vi "Koloruj wskazniki.vi"(4 "Kolor High":u32(colorbox)=16711680, 5 "High":bool, 6 "Kolor Low":u32(colorbox)=16860, 7 "Low":bool, 8 "error in (no error)":errorcluster, 11 "AI Refnum":refnum<vi>) -> (0 "error out":errorcluster)   [LabVIEW 2014]
doc: "Koloruje wskaźnik kanału analogowego nad panelem\nw zależności od zakresu ADC w zakresie/za wysoko/za nisko"
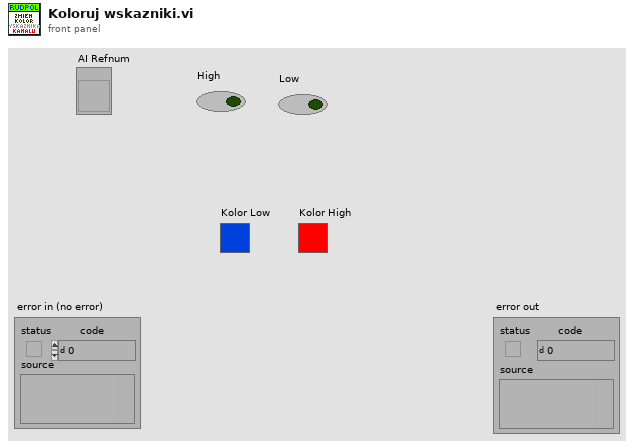
[diagram p1: front panel]
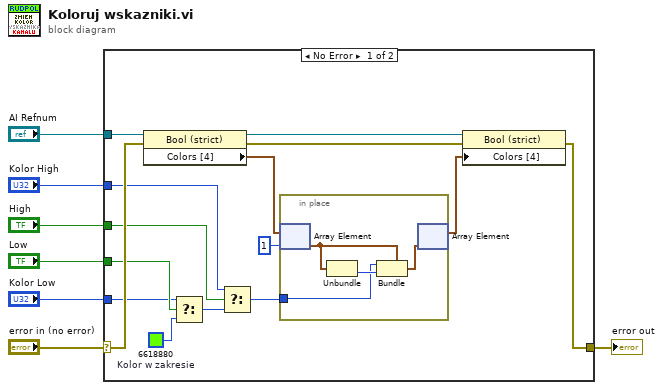
[diagram p0: block diagram]
diagram:
  n1 = case shown="No Error" "error in (no error)" {
    selector: "error in (no error)" -> [w20 w27]
    tunnel: [w19 w27] -> w6
    tunnel: "AI Refnum" -> [w22 _]
    tunnel: "Kolor Low" -> [w13 _]
    tunnel: "Kolor High" -> [w8 _]
    tunnel: "Low" -> [w14 _]
    tunnel: "High" -> [w11 _]
    frame No Error {
      w12 = u32 6618880  # Kolor w zakresie
      n2 = property class="Bool (strict)"(reference=w22, error in=w20) -> (reference out=w21:refnum<vi>, error out=w18:errorcluster, "Colors [4]"=w17:cluster{u32, u32}[])
      n3 = Select(t=w13, s=w14, f=w12) -> (s? t:f=w10:u32)
      n4 = Select(t=w8, s=w11, f=w10) -> (s? t:f=w9:u32)
      n5 = in-place {
        in-place-border: w9 -> [w23]
        n6 = in-place-array #1(w17, 1) -> (w25:cluster{u32, u32})
        n7 = Unbundle(w25) -> (w24:u32)  [unwired: 1 out]
        n8 = Bundle(cluster=w25, w23, w24) -> (w26:cluster{u32, u32})
        n9 = in-place-array #1(w26) -> (w15:cluster{u32, u32}[])  [unwired: 1 out]
      }
      n10 = property class="Bool (strict)"(reference=w21, error in=w18, "Colors [4]"=w15) -> (error out=w19:errorcluster)  [unwired: 1 out]
    }
    frame Error {
    }
  }
  "error out" <- w6
